vi "Replase ALR_ON_OFF_SharedV.vi"(10 "ALR_control":T2, 11 "ALR_ON_OFF in":refnum<data-value>) -> (3 "ALR_ON_OFF out":refnum<data-value>)   [LabVIEW 2019]
uses:
  Ctl/ALR_control_message.ctl
  Ctl/ALR_control_messages.ctl
  <vilib>/NI/Tools/Keyed Array/KeyedArray.ctl
  <vilib>/NI/Tools/Keyed Array/Tools_KeyedArray.lvlib
  Ctl/ALR_Control.ctl
  Alarms.lvlib
panel:
  in  "ALR_control":T1
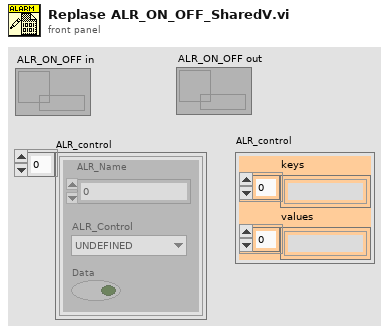
[diagram p1: front panel]
types:
  T1 = typedef "Tools_KeyedArray.lvlib/KeyedArray.ctl" = cluster{"keys":string[], "values":string[]}
  T2 = typedef "ALR_control_messages.ctl" = T3[]
  T3 = typedef "ALR_control_message.ctl" = cluster{"ALR_Name":u16, "ALR_Control":T4, "Data":bool}
  T4 = typedef "Alarms.lvlib/ALR_Control.ctl" = enum16{"UNDEFINED", "ALR_ON", "ALR_OFF", "ALR_reset", "ALR_check_ON", "ALR_reset_OFF", "ALR_check_OFF", "ALR_block_ON", "ALR_block_OFF", "ALR_Ack", "ALR_Ack_OFF"}
  T5 = cluster{"ALR_ON":bool[], "ALR_OFF":bool[], "ALR_reset":bool[], "ALR_check":bool[], "ALR_block":bool[], "ALR_Ack":bool[]}
  T6 = typedef "Alarms.lvlib/ALR_ON_OFF.ctl" = cluster{"ALR_ON":bool[], "ALR_OFF":bool[], "ALR_reset":bool[], "ALR_check":bool[], "ALR_block":bool[], "ALR_Ack":bool[]}
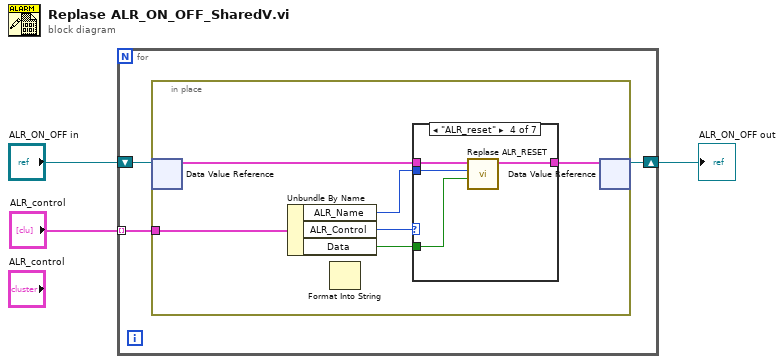
[diagram p0: block diagram]
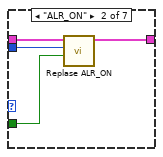
[diagram p3: hidden frame]
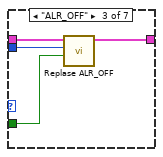
[diagram p4: hidden frame]
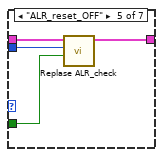
[diagram p5: hidden frame]
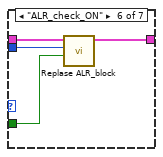
[diagram p6: hidden frame]
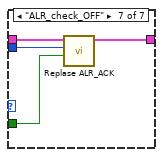
[diagram p7: hidden frame]
diagram:
  n1 = for {
    tunnel: "ALR_control" -> [w4] mode=indexing
    shift-right: [w6] -> w1
    shift-left: "ALR_ON_OFF in" -> [w5]
    n2 = in-place {
      in-place-border: w4 -> [w10]
      n3 = in-place-dvr #1(w5) -> (w12:T5)  [unwired: 1 out]
      n4 = Unbundle By Name(w10) -> ("ALR_Name"=w7:u16, "ALR_Control"=w8:T4, "Data"=w9:bool)
      n5 = Format Into String() -> ()  [unwired: 4 in, 2 out]
      n6 = case shown="\"ALR_reset\"" w8 {
        tunnel: w12 -> [w13 w17 w21 w25 w29 w33 w37]
        tunnel: [w13 w16 w20 w24 w28 w32 w36] -> w11
        tunnel: w7 -> [_ w15 w19 w23 w27 w31 w35]
        tunnel: w9 -> [_ w14 w18 w22 w26 w30 w34]
        frame "UNDEFINED", Default {
        }
        frame "ALR_ON" {
          n7 = call "Replase ALR_ON.vi"("ALR_ON"=w14, "N"=w15, "ALR_ON_OFF in"=w17) -> ("ALR_ON_OFF out"=w16:T6)  [unwired: 8 in]
        }
        frame "ALR_OFF" {
          n8 = call "Replase ALR_OFF.vi"("ALR_OFF"=w18, "N"=w19, "ALR_ON_OFF in"=w21) -> ("ALR_ON_OFF out"=w20:T6)  [unwired: 8 in]
        }
        frame "ALR_reset" {
          n9 = call "Replase ALR_RESET.vi"("ALR_RST"=w22, "N"=w23, "ALR_ON_OFF in"=w25) -> ("ALR_ON_OFF out"=w24:T6)  [unwired: 8 in]
        }
        frame "ALR_reset_OFF" {
          n10 = call "Replase ALR_check.vi"("ALR_check"=w26, "N"=w27, "ALR_ON_OFF in"=w29) -> ("ALR_ON_OFF out"=w28:T6)  [unwired: 8 in]
        }
        frame "ALR_check_ON" {
          n11 = call "Replase ALR_block.vi"("ALR_block"=w30, "N"=w31, "ALR_ON_OFF in"=w33) -> ("ALR_ON_OFF out"=w32:T6)  [unwired: 8 in]
        }
        frame "ALR_check_OFF" {
          n12 = call "Replase ALR_ACK.vi"("ALR_ACK"=w34, "N"=w35, "ALR_ON_OFF in"=w37) -> ("ALR_ON_OFF out"=w36:T6)  [unwired: 8 in]
        }
      }
      n13 = in-place-dvr #1(w11) -> (w6:refnum<data-value>)  [unwired: 1 out]
    }
  }
  "ALR_ON_OFF out" <- w1
